vi "dequeue.vi"(8 "error in (no error)":errorcluster, 11 "EventDaemon in":refnum<class "MemoryManager.lvclass">) -> (0 "error out":errorcluster, 2 "state":T1, 3 "EventDaemon out":refnum<class "MemoryManager.lvclass">, 5 "timeout":i32)   [LabVIEW 2024, in "MemoryManager.lvclass"]
doc: "Dequeues private states for daemon."
uses:
  MemoryManager.lvclass
  states--enum.ctl
  MemoryManager.lvclass/MemoryManager.ctl
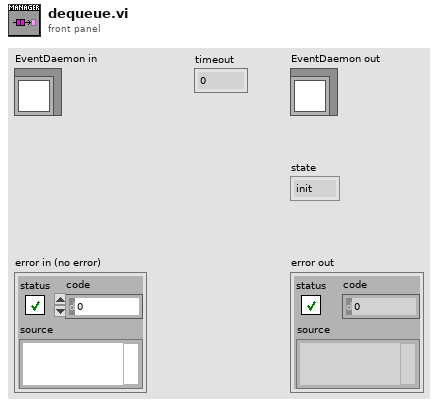
[diagram p1: front panel]
types:
  T1 = typedef "MemoryManager.lvclass/states--enum.ctl" = enum16{"init", "default", "error handler", "exit"}
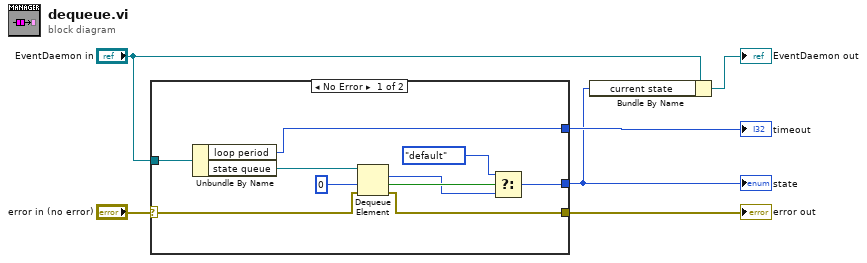
[diagram p0: block diagram]
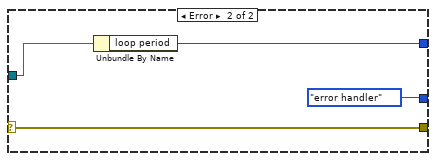
[diagram p2: hidden frame]
diagram:
  n1 = case shown="No Error" "error in (no error)" {
    selector: "error in (no error)" -> [w8 w19]
    tunnel: "EventDaemon in" -> [w16 w18]
    tunnel: [w13 w19] -> w6
    tunnel: [w9 states--enum."error handler" ("states")] -> w1
    tunnel: [w7 w17] -> w4
    frame No Error {
      n2 = Unbundle By Name(w16) -> ("loop period"=w7:i32, "state queue"=w15:refnum<queue>)
      n3 = Dequeue Element(queue=w15, timeout in ms (-1)=0, error in (no error)=w8) -> (element=w11:T1, timed out?=w12:bool, error out=w13:errorcluster)  [unwired: 1 out]
      n4 = Select(t=states--enum."default", s=w12, f=w11) -> (s? t:f=w9:T1)
    }
    frame Error {
      n5 = Unbundle By Name(w18) -> ("loop period"=w17:i32)
    }
  }
  "error out" <- w6
  "state" <- w1
  "timeout" <- w4
  n6 = Bundle By Name(cluster="EventDaemon in", "current state"=w1) -> (→"EventDaemon out":refnum<class "MemoryManager.lvclass">)
